vi "set_xml.vi"() -> ()   [LabVIEW 2010]
uses:
  <vilib>/Utility/xml.llb/Write to XML File(string).vi
panel:
  in  "XML File Path":path
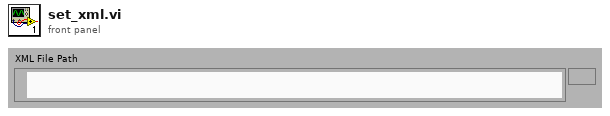
[diagram p1: front panel]
types:
  T1 = cluster{"DevNo":i32, "Cmd":string, "Param":string}
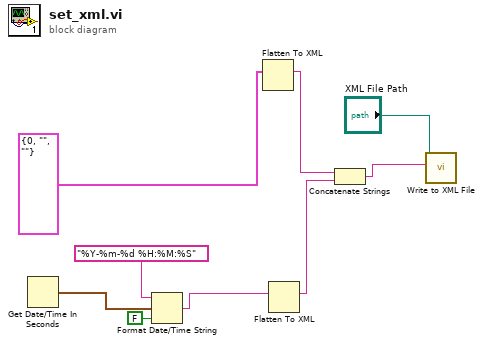
[diagram p0: block diagram]
diagram:
  n1 = Get Date/Time In Seconds() -> (seconds since 1Jan1904=w8:timestamp)
  n2 = Format Date/Time String(time format string (%c)="%Y-%m-%d %H:%M:%S", seconds (now)=w8, UTC format=FALSE) -> (date/time string=w5:string)
  n3 = Flatten To XML(anything=T1 {"DevNo"=0, "Cmd"="", "Param"=""}) -> (xml string=w4:string)
  n4 = Flatten To XML(anything=w5) -> (xml string=w3:string)
  n5 = Concatenate Strings(w4, w3) -> (w2:string)
  n6 = call-poly <vilib>:"Write to XML File.vi"("XML Input"=w2, "XML File Path"="XML File Path") -> ()  [unwired: 7 in, 3 out]
